vi "Update Fan.vi"(8 "error in (no error)":errorcluster, 9 "Fan B":T1, 10 "Fan A":T1, 11 "Cooler UI with Events in":refnum<class "Cooler UI with Events.lvclass">) -> (0 "error out":errorcluster, 3 "Cooler UI with Events out":refnum<class "Cooler UI with Events.lvclass">)   [LabVIEW 2012, in "Cooler UI.lvlib" / "Cooler UI with Events.lvclass"]
uses:
  Cooler UI with Events.lvclass
  Support/Unit Data.ctl
  Cooler UI with Events.lvclass/Cooler UI with Events.ctl
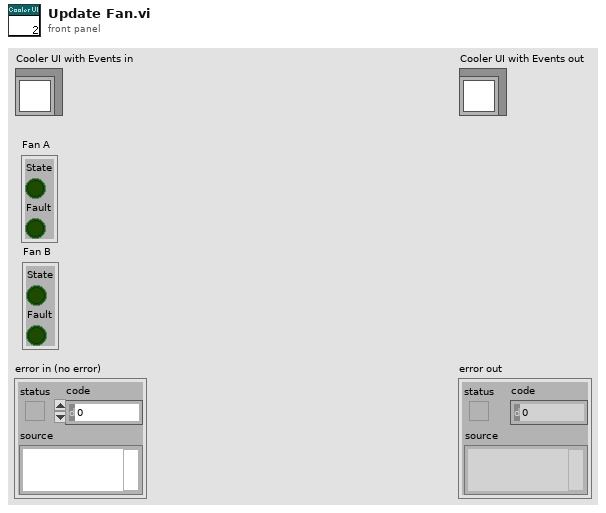
[diagram p1: front panel]
types:
  T1 = typedef "Unit Data.ctl" = cluster{"State":bool, "Fault":bool}
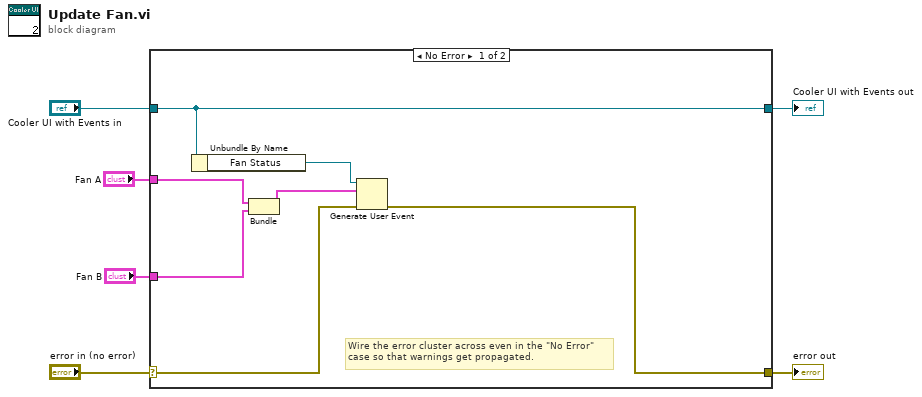
[diagram p0: block diagram]
diagram:
  n1 = case shown="No Error" "error in (no error)" {
    selector: "error in (no error)" -> [w8 w15]
    tunnel: [w7 w15] -> w5
    tunnel: [w13 w14] -> w3
    tunnel: "Cooler UI with Events in" -> [w13 w14]
    tunnel: "Fan A" -> [w9 _]
    tunnel: "Fan B" -> [w10 _]
    frame No Error {
      # "Wire the error cluster across even in the \"No Error\"\ncase so that warnings get propagated."
      n2 = Unbundle By Name(w13) -> ("Fan Status"=w12:refnum<user-event>)
      n3 = Bundle("Fan A"=w9, "Fan B"=w10) -> (w11:cluster{"Fan A":T1, "Fan B":T1})  [unwired: 1 in]
      n4 = Generate User Event(user event=w12, event data cluster=w11, error in=w8) -> (error out=w7:errorcluster)  [unwired: 1 out]
    }
    frame Error {
    }
  }
  "error out" <- w5
  "Cooler UI with Events out" <- w3
